vi "CRYPoint Clicked Check.vi"(8 "MapMode":u16(slide)=1 caption="Axis:", 9 "X-Y position of mouse":cluster{"X":dbl, "Y":dbl} {"Y" format="%.2f"; "X" format="%.2f"}, 10 "Units per pixel":cluster{"X":dbl, "Y":dbl} {"Y" format="%.2f"; "X" format="%.2f"}, 11 "Limits graph":cluster{cluster{"Hz":dbl, dbl}[]}[](array[cluster])) -> (1 "Pointer Clicked":bool, 2 "Point index":i32, 3 "Plot index":i32)   [LabVIEW 2013]
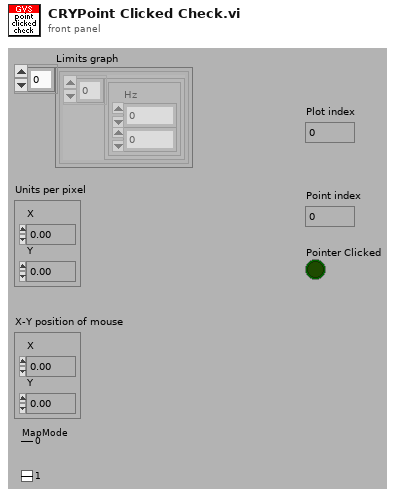
[diagram p1: front panel]
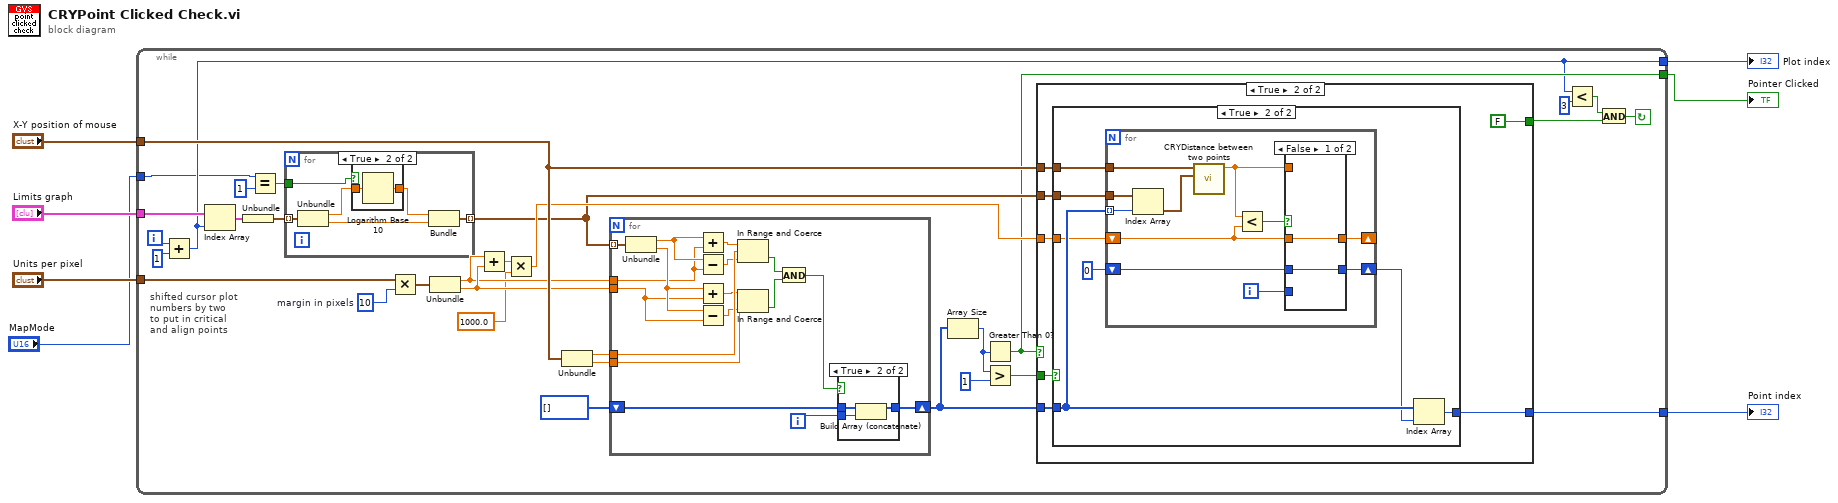
[diagram p0: block diagram]
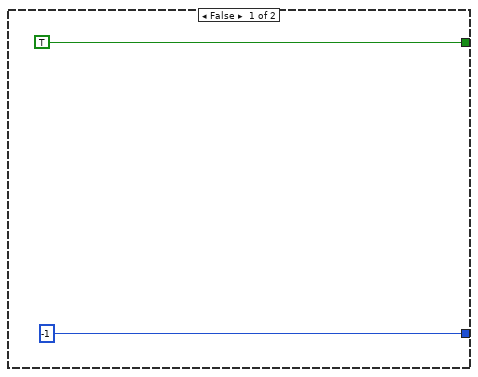
[diagram p3: hidden frame]
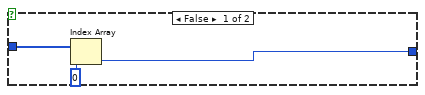
[diagram p4: hidden frame]
diagram:
  n1 = while {
    tunnel: "Units per pixel" -> [w39]
    tunnel: [w38] -> w3
    tunnel: "X-Y position of mouse" -> [w37]
    tunnel: "Limits graph" -> [w36]
    tunnel: [w11] -> w4
    tunnel: [w18] -> w5
    tunnel: "MapMode" -> [w9]
    i -> [w13]
    stop <- w16 continue-if-true
    w35 = 10  # margin in pixels
    # "shifted cursor plot numbers by two to put in critical and align points"
    n2 = Add(x=w13, y=1) -> (x+y=w11:i32)
    n3 = Index Array(array=w36, index=w11) -> (element=w21:cluster{cluster{"Hz":dbl, dbl}[]})
    n4 = Unbundle(w21) -> (w20:cluster{"Hz":dbl, dbl}[])
    n5 = Equal?(x=w9, y=u16 1) -> (x = y?=w8:bool)
    n6 = for {
      tunnel: w20 -> [w45] mode=indexing
      tunnel: [w41] -> w19 mode=indexing
      tunnel: w8 -> [w40]
      n7 = Unbundle(w45) -> ("Hz"=w43:dbl, w44:dbl)
      n8 = case shown="True" w40 {
        tunnel: w43 -> [w46 w48]
        tunnel: [w46 w47] -> w42
        frame False {
        }
        frame True {
          n9 = Logarithm Base 10(1:w48) -> (0:w47:dbl)
        }
      }
      n10 = Bundle("Hz"=w42, w44) -> (w41:cluster{"Hz":dbl, dbl})  [unwired: 1 out]
    }
    n11 = Multiply(x=w39, y=w35) -> (x*y=w34:cluster{"X":dbl, "Y":dbl})
    n12 = Unbundle(w34) -> ("X"=w25:dbl, "Y"=w26:dbl)
    n13 = Add(x=w25, y=w26) -> (x+y=w24:dbl)
    n14 = Multiply(x=w24, y=1000.0) -> (x*y=w22:dbl)
    n15 = Unbundle(w37) -> ("X"=w33:dbl, "Y"=w32:dbl)
    n16 = for {
      tunnel: w19 -> [w99] mode=indexing
      tunnel: w33 -> [w98]
      tunnel: w32 -> [w97]
      tunnel: w25 -> [w94]
      tunnel: w26 -> [w93]
      shift-right: [w84] -> w27
      shift-left: i32[] [] -> [w83]
      i -> [w85]
      n17 = Unbundle(w99) -> ("Hz"=w96:dbl, w95:dbl)
      n18 = Add(x=w96, y=w94) -> (x+y=w92:dbl)
      n19 = Subtract(x=w96, y=w94) -> (x-y=w91:dbl)
      n20 = Add(x=w95, y=w93) -> (x+y=w90:dbl)
      n21 = Subtract(x=w95, y=w93) -> (x-y=w89:dbl)
      n22 = In Range and Coerce(upper limit=w92, x=w98, lower limit=w91) -> (In Range?=w88:bool)  [unwired: 1 out]
      n23 = In Range and Coerce(upper limit=w90, x=w97, lower limit=w89) -> (In Range?=w87:bool)  [unwired: 1 out]
      n24 = And(x=w88, y=w87) -> (x .and. y?=w86:bool)
      n25 = case shown="True" w86 {
        tunnel: w85 -> [_ w103]
        tunnel: [w100 w102] -> w84
        tunnel: w83 -> [w100 w101]
        frame False {
        }
        frame True {
          n26 = Build Array (concatenate)(w101, w103) -> (w102:i32[])
        }
      }
    }
    n27 = Array Size(array=w27) -> (size(s)=w30:i32)
    n28 = Greater Than 0?(x=w30) -> (x > 0?=w18:bool)
    n29 = Greater?(x=w30, y=1) -> (0:w28:bool)
    n30 = case shown="True" w18 {
      tunnel: w28 -> [_ w57]
      tunnel: w27 -> [_ w56]
      tunnel: [-1 w55] -> w38
      tunnel: w19 -> [_ w54]
      tunnel: w37 -> [_ w53]
      tunnel: w22 -> [_ w52]
      tunnel: [TRUE FALSE] -> w17
      frame False {
      }
      frame True {
        n31 = case shown="True" w57 {
          tunnel: w56 -> [w59 w64]
          tunnel: [w58 w62] -> w55
          tunnel: w54 -> [_ w67]
          tunnel: w53 -> [_ w66]
          tunnel: w52 -> [_ w61]
          frame False {
            n32 = Index Array(array=w59, index=0 ("Index")) -> (element=w58:i32)
          }
          frame True {
            n33 = for {
              tunnel: w67 -> [w78]
              tunnel: w64 -> [w77] mode=indexing
              tunnel: w66 -> [w76]
              shift-right: [w72] -> _
              shift-left: w61 -> [w73]
              shift-right: [w70] -> w63
              shift-left: 0 -> [w71]
              i -> [w69]
              n34 = Index Array(array=w78, index=w77) -> (element=w75:cluster{"Hz":dbl, dbl})
              n35 = call "CRYDistance between two points.vi"("Point B"=w75, "Point A"=w76) -> ("Distance A to B"=w68:dbl)  [unwired: 9 out]
              n36 = Less?(x=w68, y=w73) -> (x < y?=w74:bool)
              n37 = case shown="False" w74 {
                tunnel: [w80 w82] -> w72
                tunnel: w73 -> [w80 _]
                tunnel: w71 -> [w79 _]
                tunnel: [w79 w81] -> w70
                tunnel: w68 -> [_ w82]
                tunnel: w69 -> [_ w81]
                frame False {
                }
                frame True {
                }
              }
            }
            n38 = Index Array(array=w64, index=w63) -> (element=w62:i32)
          }
        }
      }
    }
    n39 = Less?(x=w11, y=3) -> (x < y?=w14:bool)
    n40 = And(x=w14, y=w17) -> (x .and. y?=w16:bool)
  }
  "Point index" <- w3
  "Plot index" <- w4
  "Pointer Clicked" <- w5
